vi "Update Channel Count.vi"(8 "# in":u32, 9 "Array in":bool[](array[boolean]), 10 "new element/subarray":bool, 11 "Message Enqueuer":refnum<class "Message Enqueuer.lvclass">) -> (2 "Array Out":bool[](array[boolean]))   [LabVIEW 2012, in "Generic Data Logger.lvlib" / "Generic Data Logger Card.lvclass"]
uses:
  Generic Data Logger Card.lvclass
  <vilib>/ActorFramework/Message Enqueuer/Message Enqueuer.lvclass
  Generic Data Logger Card Messages/Write Array of Channel Control Msg/Write Array of Channel Control Msg.lvclass/Write Array of Channel Control Msg.ctl
  <vilib>/ActorFramework/Message Enqueuer/Message Enqueuer.lvclass/Message Enqueuer.ctl
  <vilib>/ActorFramework/Message Enqueuer/Enqueue.vi
  <vilib>/ActorFramework/Message Priority Queue/Priority Enqueue.vi
  Generic Data Logger Card Messages/Write Array of Channel Control Msg/Write Array of Channel Control Msg.lvclass
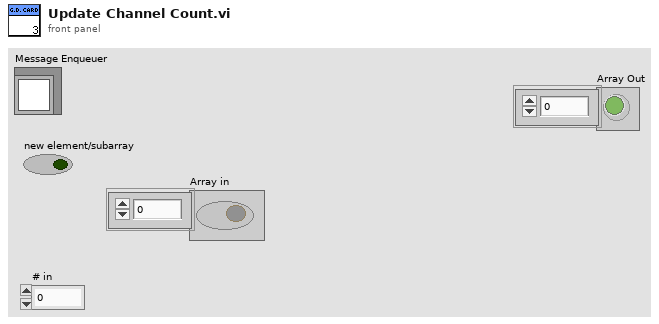
[diagram p1: front panel]
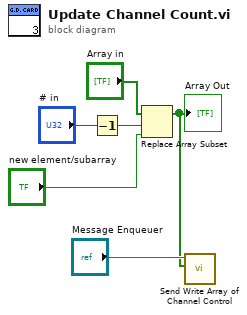
[diagram p0: block diagram]
diagram:
  n1 = Decrement(x="# in") -> (x-1=w5:u32)
  n2 = Replace Array Subset(array="Array in", new element="new element/subarray", index=w5) -> (w1:bool[])
  "Array Out" <- w1
  n3 = call "Send Write Array of Channel Control.vi"("Array in"=w1, "Message Enqueuer"="Message Enqueuer") -> ()  [unwired: 8 in, 2 out]
